vi "Write SerialCommunicator.vi"(8 "error in (no error)":errorcluster, 10 "SerialProtocols.lvlib:SerialCommunicator.lvclass":refnum<class "SerialCommunicator.lvclass">, 11 "SerialClient in":refnum<class "SerialCommunication.lvclass">) -> (0 "error out":errorcluster, 3 "SerialClient out":refnum<class "SerialCommunication.lvclass">)   [LabVIEW 2016, in "SerialCommunication.lvclass"]
uses:
  SerialCommunication.lvclass
  common_serialprotocols/SerialCommunicator/SerialCommunicator.lvclass
  SerialCommunication.lvclass/SerialCommunication.ctl
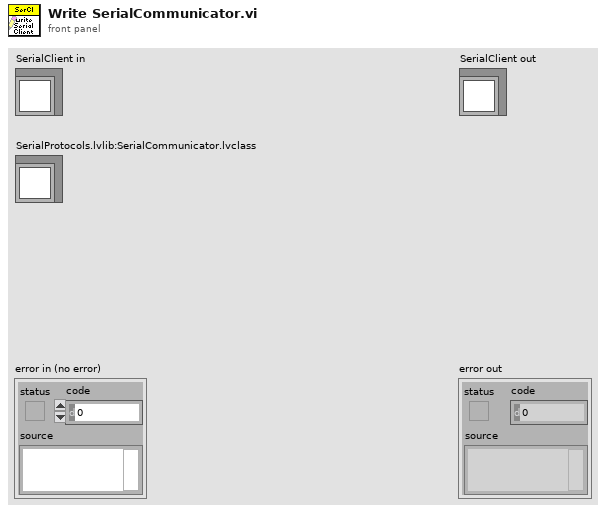
[diagram p1: front panel]
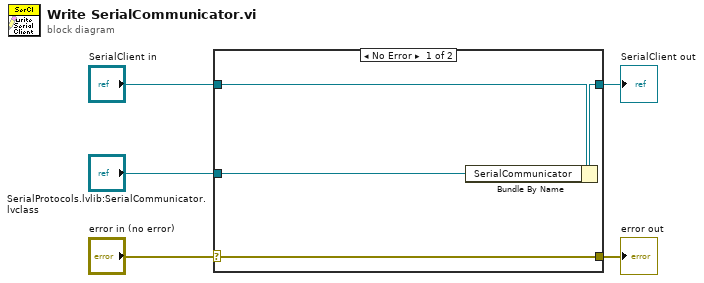
[diagram p0: block diagram]
diagram:
  n1 = case shown="No Error" "error in (no error)" {
    selector: "error in (no error)" -> [w9 w10]
    tunnel: [w9 w10] -> w4
    tunnel: [w7 w11] -> w2
    tunnel: "SerialClient in" -> [w8 w11]
    tunnel: "SerialProtocols.lvlib:SerialCommunicator.lvclass" -> [w6 _]
    frame No Error {
      n2 = Bundle By Name(cluster=w8, "SerialCommunicator"=w6) -> (w7:refnum<class "SerialCommunication.lvclass">)
    }
    frame Error {
    }
  }
  "error out" <- w4
  "SerialClient out" <- w2
